vi "RenderRobotPose.vi"(0 "Robot X (in)":dbl, 1 "Robot Width (in)":dbl=30.0 format="%#_13g", 2 "Robot Length (in)":dbl=30.0 format="%#_13g", 3 "Buffer Time (min)":dbl=5.0 format="%#_13g", 5 "Robot Y (in)":dbl, 7 "Targeting Information":dbl[](array[numeric])=[0.0, 0.0, 0.0, 0.0], 9 "Robot Heading (deg)":dbl, 11 "Planned Path":T1, 12 "Robot Enabled":bool, 14 "Reset":bool) -> (6 "Robot Pose":cluster{dbl[], dbl[]}[](graph))   [LabVIEW 2023]
doc: "This VI takes the robot pose information as input and renders a plot to display it. At this time, only square robot dimensions are supported."
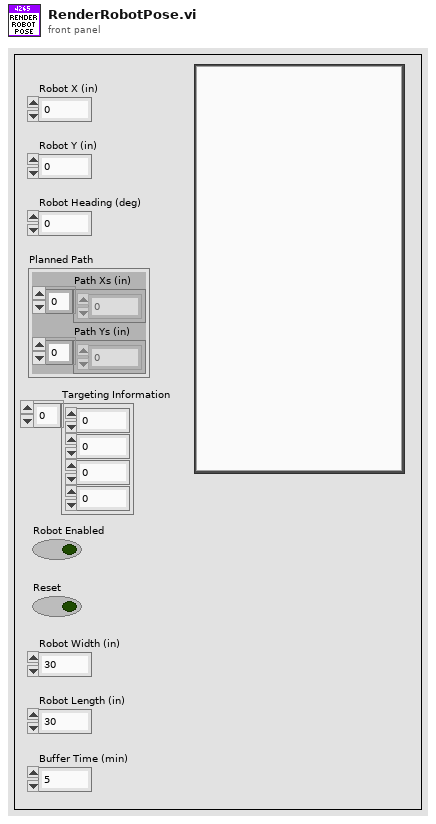
[diagram p1: front panel]
types:
  T1 = cluster{"Path Xs (in)":dbl[], "Path Ys (in)":dbl[]}
  T2 = cluster{"Path Xs (in)":dbl[], "Path Ys (in)":dbl[]}[]
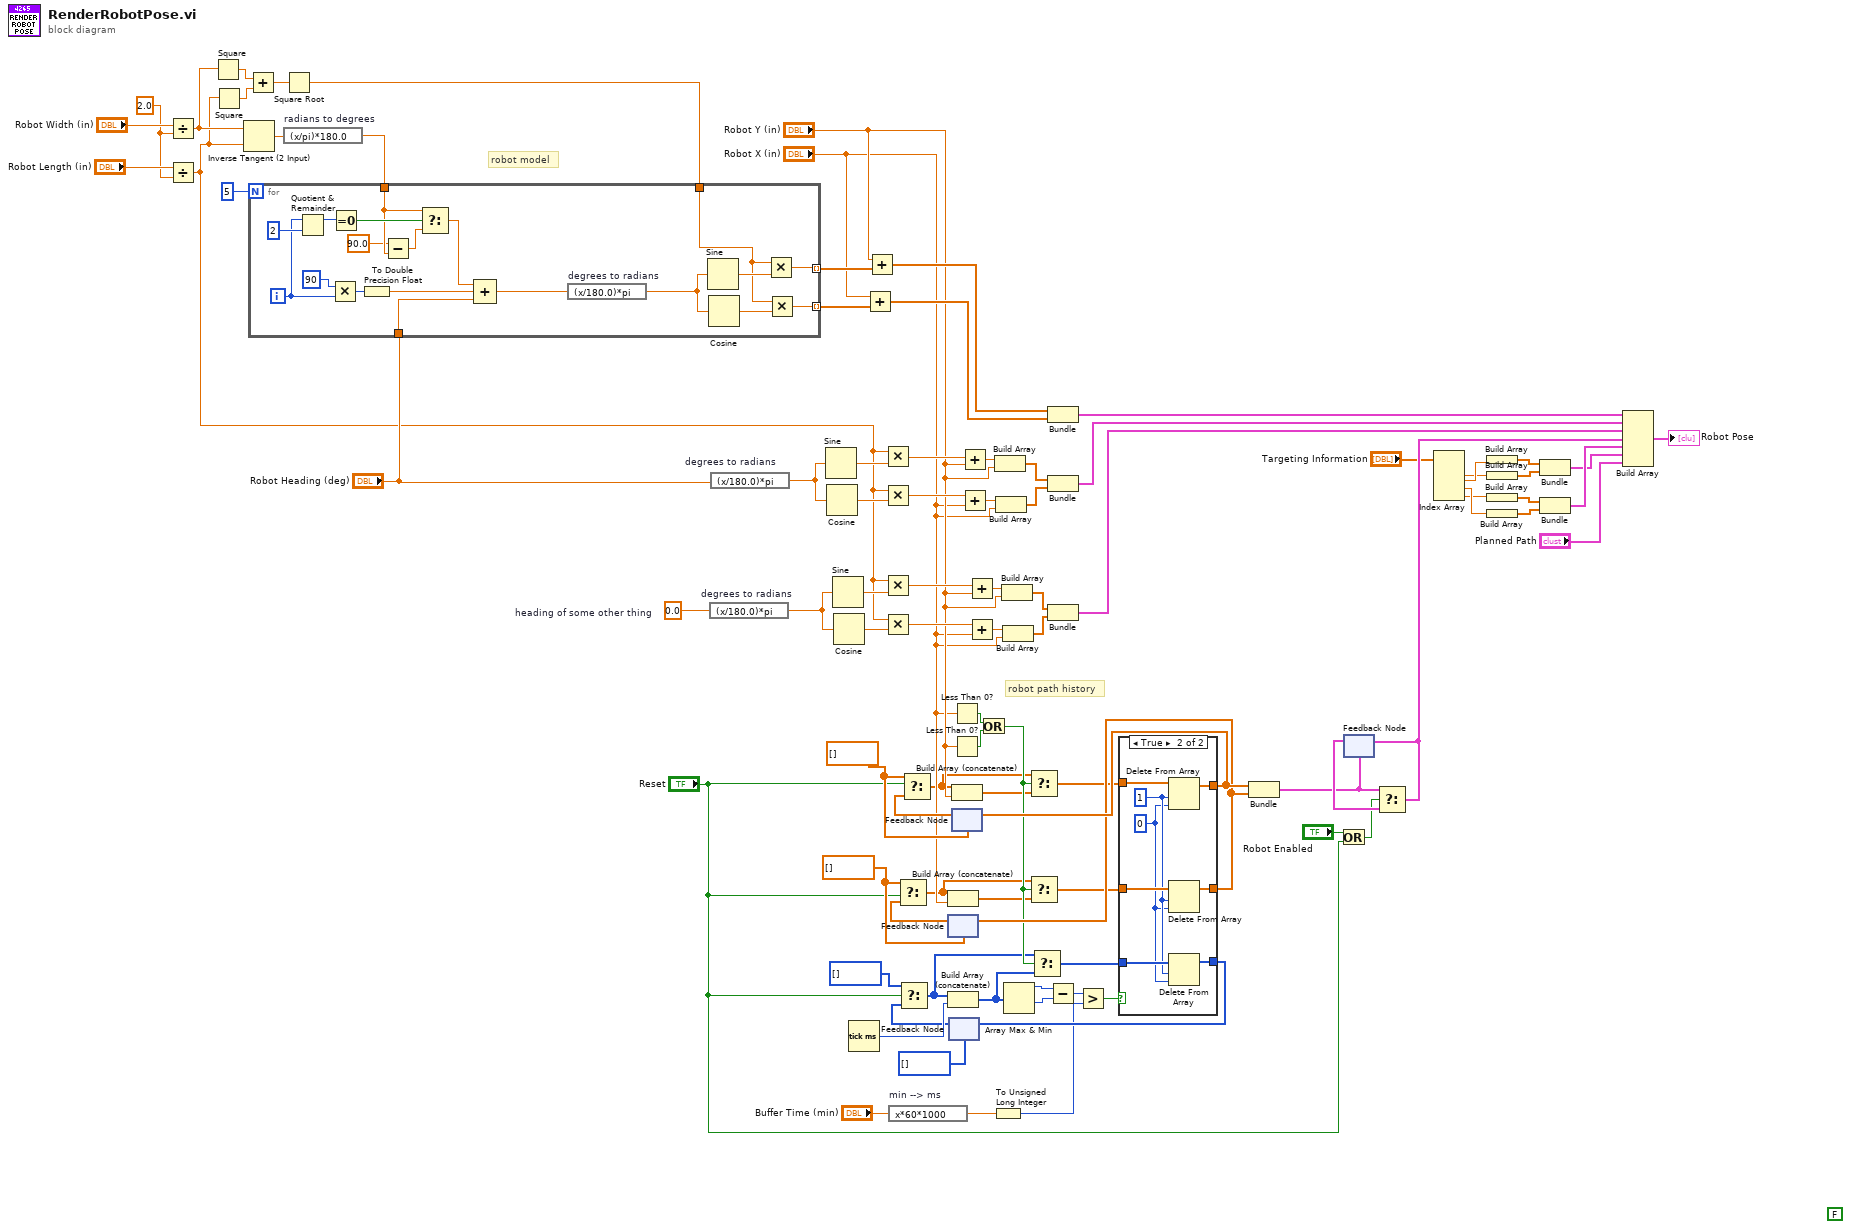
[diagram p0: block diagram]
diagram:
  w4 = 0.0  # heading of some other thing
  w22 = 2.0
  (unwired) FALSE
  w41 = dbl[] [] ("t")
  w40 = dbl[] [] ("t")
  # "robot model"
  # "robot path history"
  n1 = Divide(x="Robot Width (in)", y=w22) -> (x/y=w19:dbl)
  n2 = Divide(x="Robot Length (in)", y=w22) -> (x/y=w18:dbl)
  n3 = Square(x=w19) -> (x^2=w16:dbl)
  n4 = Square(x=w18) -> (x^2=w17:dbl)
  n5 = Inverse Tangent (2 Input)(1:w18, 2:w19) -> (0:w21:dbl)
  n6 = Add(x=w16, y=w17) -> (x+y=w15:dbl)
  n7 = Square Root(x=w15) -> (sqrt(x)=w14:dbl)
  n8 = expression code="(x/pi)*180.0" "radians to degrees"(w21) -> (w20:dbl)
  n9 = for {
    N: 5 -> [_]
    tunnel: [w106] -> w89 mode=indexing
    tunnel: [w105] -> w88 mode=indexing
    tunnel: "Robot Heading (deg)" -> [w100]
    tunnel: w20 -> [w96]
    tunnel: w14 -> [w91]
    i -> [w92]
    n10 = Quotient & Remainder(x=w92, y=2) -> (x-y*floor(x/y)=w98:i32)  [unwired: 1 out]
    n11 = Multiply(x=90, y=w92) -> (x*y=w103:i32)
    n12 = Equal To 0?(x=w98) -> (x = 0?=w97:bool)
    n13 = To Double Precision Float(number=w103) -> (double precision float=w102:dbl)
    n14 = Subtract(x=90.0, y=w96) -> (x-y=w95:dbl)
    n15 = Select(t=w96, s=w97, f=w95) -> (s? t:f=w93:dbl)
    n16 = Compound Arithmetic op=ADD(w93, w102, w100) -> (w101:dbl)
    n17 = expression code="(x/180.0)*pi" "degrees to radians"(w101) -> (w108:dbl)
    n18 = Sine(x=w108) -> (sin(x)=w107:dbl)
    n19 = Cosine(x=w108) -> (cos(x)=w109:dbl)
    n20 = Multiply(x=w91, y=w107) -> (x*y=w105:dbl)
    n21 = Multiply(x=w91, y=w109) -> (x*y=w106:dbl)
  }
  n22 = expression code="(x/180.0)*pi" "degrees to radians"(w4) -> (w66:dbl)
  n23 = expression code="(x/180.0)*pi" "degrees to radians"("Robot Heading (deg)") -> (w55:dbl)
  n24 = Sine(x=w55) -> (sin(x)=w54:dbl)
  n25 = Cosine(x=w55) -> (cos(x)=w53:dbl)
  n26 = Sine(x=w66) -> (sin(x)=w65:dbl)
  n27 = Cosine(x=w66) -> (cos(x)=w64:dbl)
  n28 = Tick Count (ms)() -> (millisecond timer value=w72:u32)
  n29 = Add(x="Robot X (in)", y=w89) -> (x+y=w86:dbl[])
  n30 = Add(x="Robot Y (in)", y=w88) -> (x+y=w85:dbl[])
  n31 = Multiply(x=w18, y=w54) -> (x*y=w52:dbl)
  n32 = Multiply(x=w18, y=w53) -> (x*y=w51:dbl)
  n33 = Multiply(x=w18, y=w65) -> (x*y=w63:dbl)
  n34 = Multiply(x=w18, y=w64) -> (x*y=w62:dbl)
  n35 = expression code="x*60*1000" "min --> ms"("Buffer Time (min)") -> (w77:dbl)
  n36 = feedback #1(w40) -> (w68:dbl[])
  n37 = Select(t=w40, s="Reset", f=w68) -> (s? t:f=w29:dbl[])
  n38 = Build Array (concatenate)(w29, "Robot X (in)") -> (w30:dbl[])
  n39 = feedback #2(u32[] []) -> (w70:u32[])
  n40 = Select(t=u32[] [], s="Reset", f=w70) -> (s? t:f=w34:u32[])
  n41 = Build Array (concatenate)(w34, w72) -> (w33:u32[])
  n42 = Less Than 0?(x="Robot X (in)") -> (x < 0?=w37:bool)
  n43 = Less Than 0?(x="Robot Y (in)") -> (x < 0?=w38:bool)
  n44 = feedback #3(w41) -> (w71:dbl[])
  n45 = Select(t=w41, s="Reset", f=w71) -> (s? t:f=w31:dbl[])
  n46 = Build Array (concatenate)(w31, "Robot Y (in)") -> (w32:dbl[])
  n47 = Add(x=w52, y="Robot Y (in)") -> (x+y=w50:dbl)
  n48 = Add(x=w51, y="Robot X (in)") -> (x+y=w49:dbl)
  n49 = Add(x=w63, y="Robot Y (in)") -> (x+y=w61:dbl)
  n50 = Add(x=w62, y="Robot X (in)") -> (x+y=w60:dbl)
  n51 = Or(x=w37, y=w38) -> (x .or. y?=w36:bool)
  n52 = To Unsigned Long Integer(number=w77) -> (unsigned 32bit integer=w78:u32)
  n53 = Build Array(w50, "Robot Y (in)") -> (w48:dbl[])
  n54 = Build Array(w49, "Robot X (in)") -> (w47:dbl[])
  n55 = Build Array(w61, "Robot Y (in)") -> (w59:dbl[])
  n56 = Build Array(w60, "Robot X (in)") -> (w58:dbl[])
  n57 = Array Max & Min(array=w33) -> (max value=w74:u32, min value=w75:u32)  [unwired: 2 out]
  n58 = Select(t=w31, s=w36, f=w32) -> (s? t:f=w43:dbl[])
  n59 = Select(t=w29, s=w36, f=w30) -> (s? t:f=w42:dbl[])
  n60 = Select(t=w34, s=w36, f=w33) -> (s? t:f=w35:u32[])
  n61 = Bundle(w85, w86) -> (w57:cluster{dbl[], dbl[]})  [unwired: 1 in]
  n62 = Bundle(w48, w47) -> (w56:cluster{dbl[], dbl[]})  [unwired: 1 in]
  n63 = Bundle(w59, w58) -> (w67:cluster{dbl[], dbl[]})  [unwired: 1 in]
  n64 = Subtract(x=w74, y=w75) -> (x-y=w76:u32)
  n65 = Greater?(x=w76, y=w78) -> (0:w80:bool)
  n66 = case shown="True" w80 {
    tunnel: w35 -> [w110 w118]
    tunnel: w42 -> [w111 w119]
    tunnel: w43 -> [w112 w120]
    tunnel: [w112 w115] -> w83
    tunnel: [w111 w114] -> w82
    tunnel: [w110 w113] -> w81
    frame False {
    }
    frame True {
      w116 = 0 ("index")
      w117 = 1 ("length")
      n67 = Delete From Array(array=w120, length=w117, index=w116) -> (array with subset deleted=w115:dbl[])  [unwired: 1 out]
      n68 = Delete From Array(array=w119, length=w117, index=w116) -> (array with subset deleted=w114:dbl[])  [unwired: 1 out]
      n69 = Delete From Array(array=w118, length=w117, index=w116) -> (array with subset deleted=w113:u32[])  [unwired: 1 out]
    }
  }
  n70 = feedback-in #1(w82) -> ()
  n71 = feedback-in #2(w81) -> ()
  n72 = feedback-in #3(w83) -> ()
  n73 = Bundle("t"=w83, "t"=w82) -> (w46:cluster{"t":dbl[], "t":dbl[]})  [unwired: 1 in]
  n74 = Or(x="Robot Enabled", y="Reset") -> (x .or. y?=w26:bool)
  n75 = feedback #4(w46) -> (w84:cluster{"t":dbl[], "t":dbl[]})
  n76 = Select(t=w46, s=w26, f=w84) -> (s? t:f=w45:cluster{"t":dbl[], "t":dbl[]})
  n77 = feedback-in #4(w45) -> ()
  n78 = Index Array(array="Targeting Information") -> (element #1=w7:dbl, element #2=w8:dbl, element #3=w6:dbl, element #4=w5:dbl)  [unwired: 4 in]
  n79 = Build Array(w8) -> (w13:dbl[])
  n80 = Build Array(w7) -> (w12:dbl[])
  n81 = Build Array(w5) -> (w11:dbl[])
  n82 = Build Array(w6) -> (w10:dbl[])
  n83 = Bundle(w13, w12) -> (w2:cluster{dbl[], dbl[]})  [unwired: 1 in]
  n84 = Bundle(w11, w10) -> (w3:cluster{dbl[], dbl[]})  [unwired: 1 in]
  n85 = Build Array(w57, w56, w67, w45, w3, w2, "Planned Path") -> (→"Robot Pose":T2)
